vi "Set Control Font.vi"(4 "Error In":errorcluster, 6 "Font Parameters":T1, 7 "Font Settting in":refnum<class "Display Properties_Boolean.lvclass">) -> (0 "Error Out":errorcluster, 3 "Font Settting out":refnum<class "Display Properties_Boolean.lvclass">)   [LabVIEW 2015, in "Display Properties Manager.lvlib" / "Display Properties_Boolean.lvclass"]
uses:
  Display Properties_Boolean.lvclass
  _typedefs/Font Parameters.ctl
  _typedefs/Control Component to Set.ctl
  Display Properties.lvclass
  Display Properties Manager.lvlib
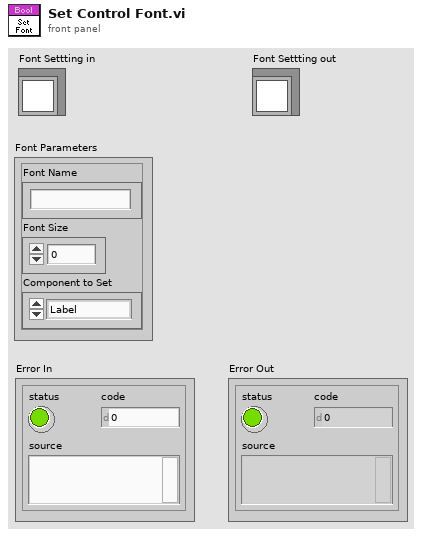
[diagram p1: front panel]
types:
  T1 = typedef "Display Properties Manager.lvlib/Font Parameters.ctl" = cluster{"Font Name":string, "Font Size":u32, "Component to Set":T2}
  T2 = typedef "Display Properties Manager.lvlib/Control Component to Set.ctl" = enum16{"Label", "Caption", "Contents"}
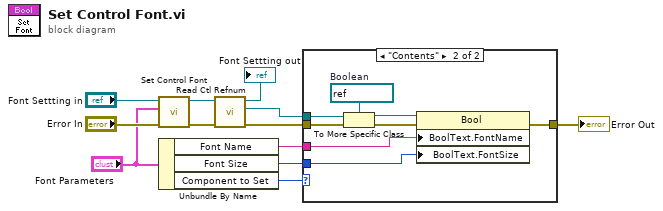
[diagram p0: block diagram]
diagram:
  n1 = call-parent "Set Control Font.vi"("Error In"="Error In", "Font Parameters"="Font Parameters", "Font Settting in"="Font Settting in") -> ("Error Out"=w9:errorcluster, "Font Settting out"=w10:refnum<class "Display Properties_Boolean.lvclass">)  [unwired: 3 in]
  n2 = Unbundle By Name("Font Parameters") -> ("Font Name"=w2:string, "Font Size"=w1:u32, "Component to Set"=w4:T2)
  n3 = call-dynamic "Read Ctl Refnum.vi"("Error In"=w9, "Font Settting in"=w10) -> ("Error Out"=w7:errorcluster, "Ctl Refnum"=w3:refnum<vi>, "Font Settting out"=→"Font Settting out":refnum<class "Display Properties_Boolean.lvclass">)  [unwired: 3 in]
  n4 = case shown="\"Contents\"" w4 {
    tunnel: w7 -> [w13 w21]
    tunnel: [w13 w20] -> w6
    tunnel: w3 -> [_ w18]
    tunnel: w2 -> [_ w15]
    tunnel: w1 -> [_ w14]
    frame Default {
    }
    frame "Contents" {
      w16 = refnum<vi> refnum  # Boolean
      n5 = To More Specific Class(target class=w16, reference=w18, error in=w21) -> (specific class reference=w17:refnum<vi>, error out=w19:errorcluster)
      n6 = property class="Bool"(reference=w17, error in=w19, "BoolText.FontName"=w15, "BoolText.FontSize"=w14) -> (error out=w20:errorcluster)  [unwired: 1 out]
    }
  }
  "Error Out" <- w6
